vi "S7-TCP_OPEN.vi"(7 "Port":u16=102, 8 "error in (no error)":errorcluster caption="错误输入（无错误）", 9 "PLC":u8(ring)=2 items=["S7-1200.200SMART"=0, "S7-300"=2, "S7-400"=3], 10 "IP Address":string="127.0.0.1", 11 "S7-TCP 输入":refnum<class "S7-TCP.lvclass">) -> (0 "error out":errorcluster caption="错误输出", 2 "Successful？":bool, 3 "S7-TCP 输出":refnum<class "S7-TCP.lvclass">)   [LabVIEW 2018, in "S7-TCP.lvclass"]
uses:
  S7-TCP.lvclass
  S7-TCP.lvclass/S7-TCP.ctl
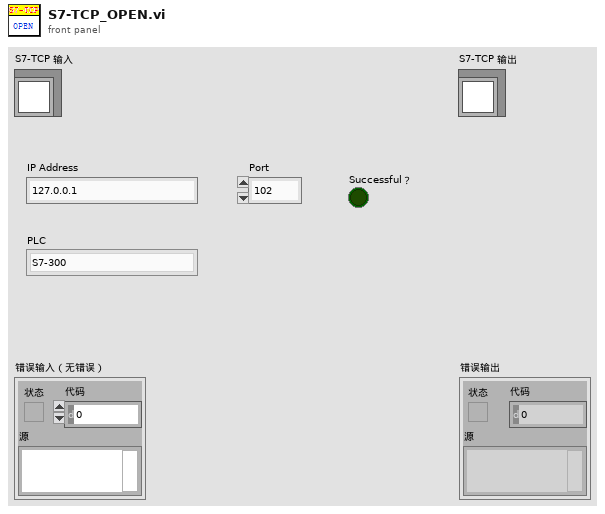
[diagram p1: front panel]
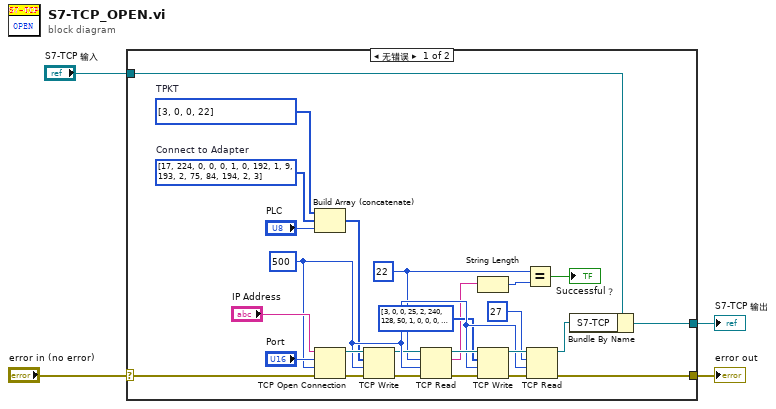
[diagram p0: block diagram]
diagram:
  n1 = case shown="无错误" "error in (no error)" {
    selector: "error in (no error)" -> [w6 w32]
    tunnel: [w5 w32] -> w3
    tunnel: [w8 w31] -> w1
    tunnel: "S7-TCP 输入" -> [w9 w31]
    frame No Error {
      w21 = 500 ("超时（MS）")
      w16 = u8[] [17, 224, 0, 0, 0, 1, 0, 192, 1, 9, 193, 2, 75, 84, 194, 2, 3]  # Connect to Adapter
      w13 = 22 ("bytes to read")
      w17 = u8[] [3, 0, 0, 22]  # TPKT
      n2 = Build Array (concatenate)(w17, w16, "PLC") -> (w12:u8[])
      n3 = TCP Open Connection(address="IP Address", remote port or service name="Port", timeout ms (60000)=w21, error in (no error)=w6) -> (connection ID=w25:refnum<k5>, error out=w24:errorcluster)  [unwired: 1 out]
      n4 = TCP Write(connection ID=w25, data in=w12, error in (no error)=w24, 9:w21) -> (connection ID out=w19:refnum<k5>, error out=w18:errorcluster)  [unwired: 1 out]
      n5 = TCP Read(connection ID=w19, bytes to read=w13, error in (no error)=w18, 9:w21) -> (connection ID out=w23:refnum<k5>, data out=w15:string, error out=w22:errorcluster)  [unwired: 1 in]
      n6 = String Length(string=w15) -> (length=w14:i32)
      n7 = TCP Write(connection ID=w23, data in=u8[] [3, 0, 0, 25, 2, 240, 128, 50, 1, 0, 0, 0, 13, 0, 8, 0, 0, 240, 0, 0, 1, 0, 1, 0, 240] ("添加的数组"), error in (no error)=w22, 9:w21) -> (connection ID out=w28:refnum<k5>, error out=w27:errorcluster)  [unwired: 1 out]
      n8 = Equal?(x=w13, y=w14) -> (x = y?=→"Successful？":bool)
      n9 = TCP Read ("读取TCP数据")(connection ID=w28, bytes to read=27 ("读取的字节"), error in (no error)=w27, 9:w21) -> (connection ID out=w7:refnum<k5>, error out=w5:errorcluster)  [unwired: 1 in, 1 out]
      n10 = Bundle By Name(cluster=w9, "S7-TCP"=w7) -> (w8:refnum<class "S7-TCP.lvclass">)
    }
    frame Error {
    }
  }
  "error out" <- w3
  "S7-TCP 输出" <- w1
